vi "SelectSignals.vi"(8 "error in (no error)":errorcluster caption="Error in", 11 "DevicesAndSignals":T1) -> (0 "error out":errorcluster caption="Error out", 2 "Cancel":bool, 3 "DevicesAndSignals":T1)   [LabVIEW 2016]
doc: "Select certain signals that should be used later (e.g. for measuring).\n\nDevicesAndSignals (Input): Cluster consisting of an array of devices and an array of signals.\nDevicesAndSignals (Output): Cluster consisting of an array of devices and an array of SELECTED signals."
panel:
  in  "AdoptSelectedSignals":bool
  in  "Cancel":bool
  in  "tvAvailableSignals":string(tree)
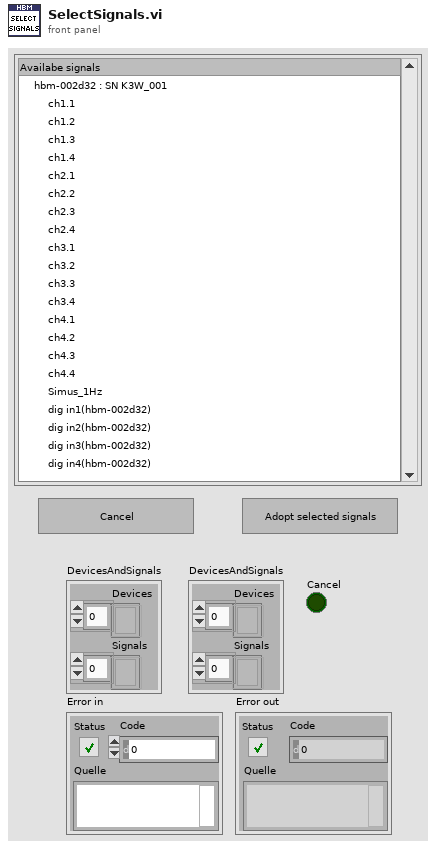
[diagram p1: front panel]
types:
  T1 = cluster{"Devices":refnum<k24>[], "Signals":refnum<k24>[]}
  T2 = typedef "LVPoint32TypeDef.ctl" = cluster{"Horizontal":i32, "Vertical":i32}
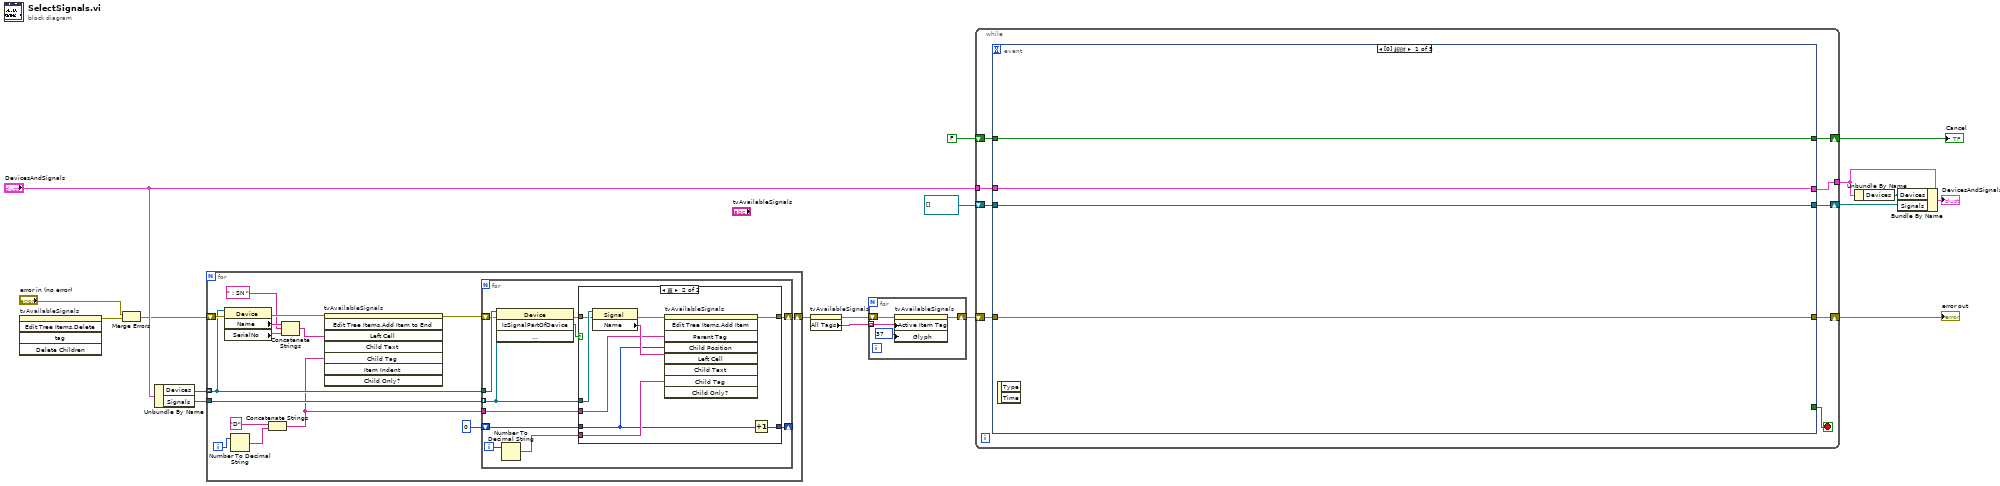
[diagram p0: block diagram]
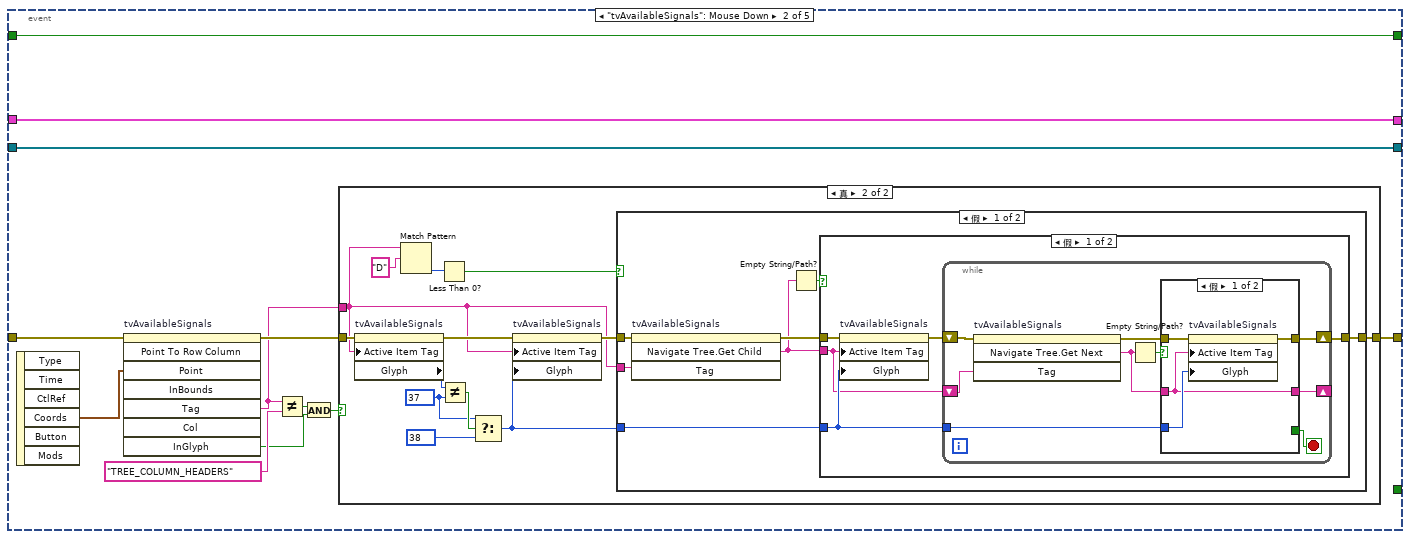
[diagram p3: hidden frame]
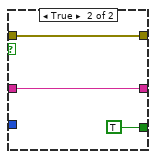
[diagram p5: hidden frame]
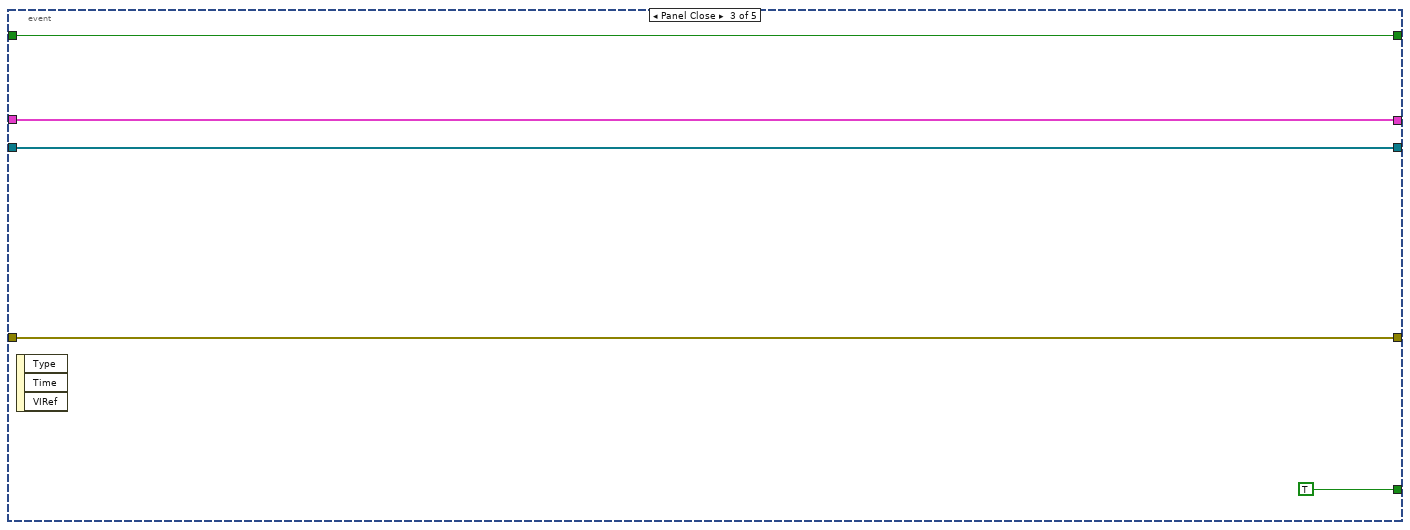
[diagram p8: hidden frame]
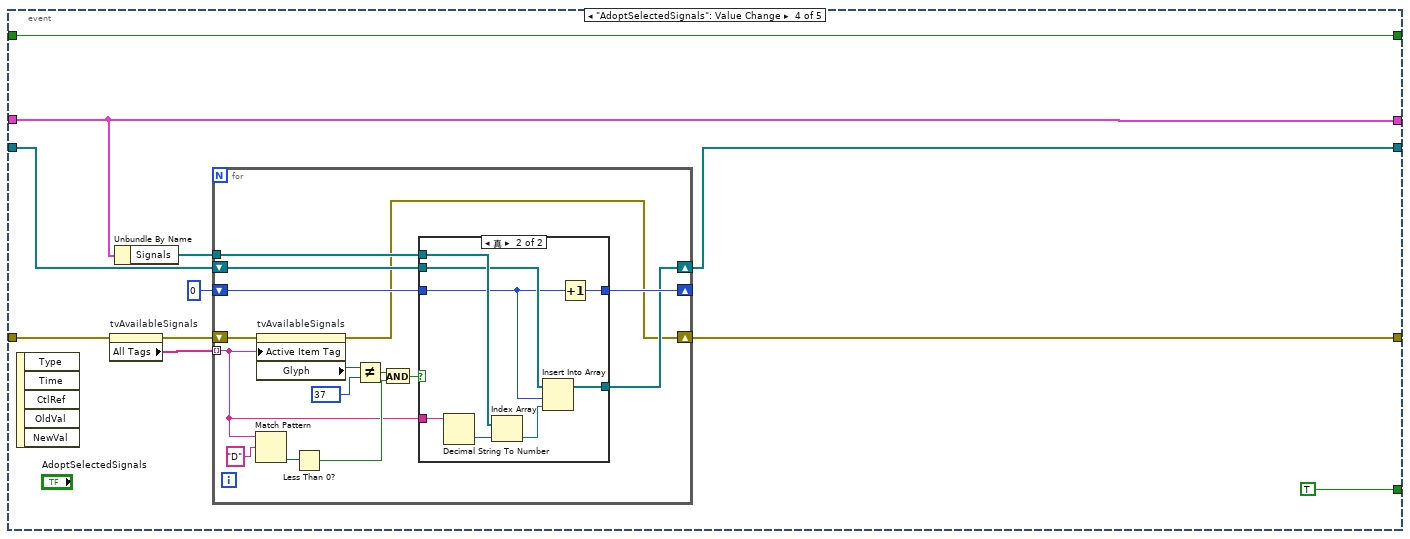
[diagram p9: hidden frame]
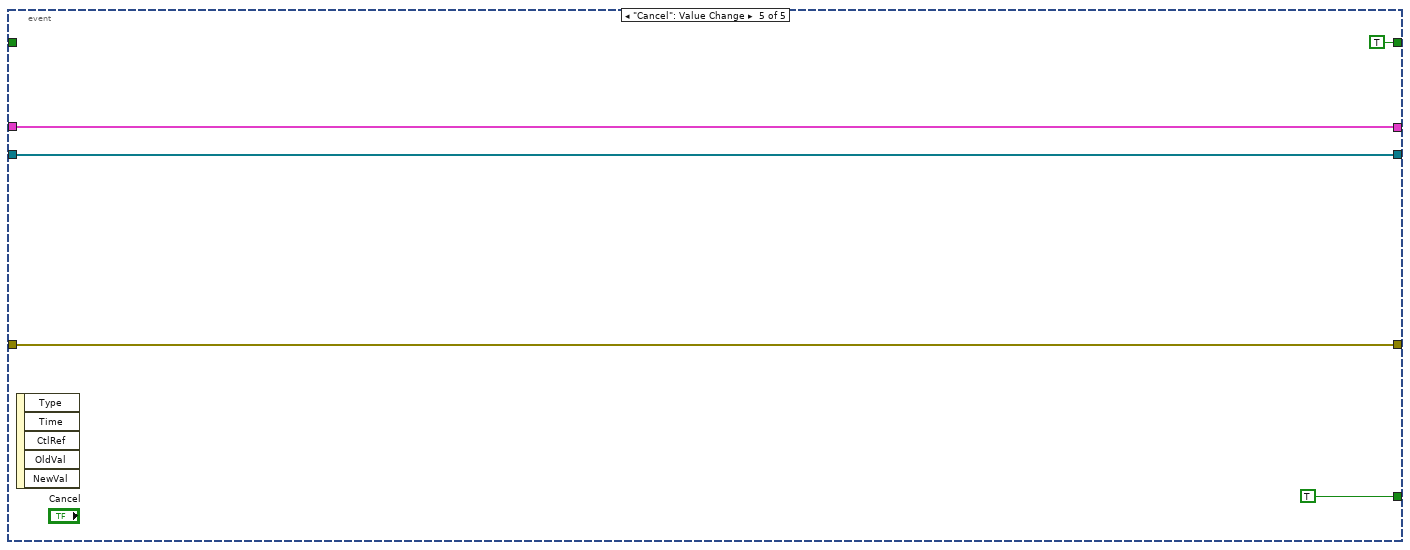
[diagram p11: hidden frame]
diagram:
  n1 = invoke on="tvAvailableSignals" class="Baum (strikt)" method="Edit Tree Items.Delete"() -> (error out=w5:errorcluster)  [unwired: 5 in, 4 out]
  n2 = Merge Errors("error in (no error)", w5) -> (w3:errorcluster)
  n3 = Unbundle By Name("DevicesAndSignals") -> ("Devices"=w14:refnum<k24>[], "Signals"=w13:refnum<k24>[])
  n4 = for {
    tunnel: w14 -> [w25] mode=indexing
    tunnel: w13 -> [w33]
    shift-right: [w19] -> w12
    shift-left: w3 -> [w31]
    i -> [w32]
    n5 = property on="Eigenschaftsknoten" class="Device"(reference=w25, error in=w31) -> (error out=w30:errorcluster, "Name"=w29:string, "SerialNo"=w28:string)  [unwired: 1 out]
    n6 = Number To Decimal String(number=w32) -> (decimal integer string=w23:string)  [unwired: 1 in]
    n7 = Concatenate Strings("D" ("String"), w23) -> (w22:string)
    n8 = Concatenate Strings(w29, " : SN " ("String"), w28) -> (w26:string)
    n9 = invoke on="tvAvailableSignals" class="Baum (strikt)" method="Edit Tree Items.Add Item to End"(error in=w30, "Left Cell"=w26, "Child Tag"=w22) -> (error out=w24:errorcluster)  [unwired: 5 in, 7 out]
    n10 = for {
      tunnel: w25 -> [w44]
      tunnel: w33 -> [w40] mode=indexing
      tunnel: w22 -> [w39]
      shift-right: [w35] -> _
      shift-left: 0 -> [w36]
      shift-right: [w34] -> w19
      shift-left: w24 -> [w42]
      i -> [w38]
      n11 = invoke on="Methodenknoten" class="Device" method="IsSignalPartOfDevice"(reference=w44, error in=w42, "signalToCheck"=w40) -> (error out=w41:errorcluster, "IsSignalPartOfDevice"=w43:bool)  [unwired: 1 in, 2 out]
      n12 = Number To Decimal String(number=w38) -> (decimal integer string=w37:string)  [unwired: 1 in]
      n13 = case shown="真" w43 {
        tunnel: w41 -> [w45 w54]
        tunnel: w40 -> [_ w55]
        tunnel: w39 -> [_ w51]
        tunnel: w37 -> [_ w50]
        tunnel: w36 -> [w46 w48]
        tunnel: [w46 w49] -> w35
        tunnel: [w45 w47] -> w34
        frame False {
        }
        frame True {
          n14 = property on="Eigenschaftsknoten" class="Signal"(reference=w55, error in=w54) -> (error out=w52:errorcluster, "Name"=w53:string)  [unwired: 1 out]
          n15 = invoke on="tvAvailableSignals" class="Baum (strikt)" method="Edit Tree Items.Add Item"(error in=w52, "Parent Tag"=w51, "Child Position"=w48, "Left Cell"=w53, "Child Tag"=w50) -> (error out=w47:errorcluster)  [unwired: 4 in, 8 out]
          n16 = Increment(x=w48) -> (x+1=w49:i32)
        }
      }
    }
  }
  n17 = property on="tvAvailableSignals" class="Tree (严格)"(error in=w12) -> (error out=w16:errorcluster, "All Tags"=w17:string[])  [unwired: 1 in, 1 out]
  n18 = for {
    tunnel: w17 -> [w59] mode=indexing
    shift-right: [w56] -> w15
    shift-left: w16 -> [w57]
    n19 = property on="tvAvailableSignals" class="Tree (严格)"(error in=w57, "Active Item Tag"=w59, "Glyph"=37) -> (error out=w56:errorcluster)  [unwired: 1 in, 1 out]
  }
  n20 = while {
    shift-right: [w66] -> w18
    shift-left: w15 -> [w67]
    shift-right: [w63] -> w7
    shift-left: refnum<k24>[] [] ("Signals") -> [w65]
    tunnel: "DevicesAndSignals" -> [w64]
    tunnel: [w62] -> w9
    shift-right: [w60] -> w1
    shift-left: FALSE -> [w61]
    stop <- w68 stop-if-true
    n21 = event shown="[0] 超时" {
      selector: _ -> [_ _ _ _ _]
      dyn-events: _ -> [_ _ _ _ _]
      timeout: _ -> [_ _ _ _ _]
      tunnel: [_ _ TRUE TRUE TRUE] -> w68
      tunnel: w67 -> [w72 w83 w130 w144 w173]
      tunnel: [w72 w81 w130 w136 w173] -> w66
      tunnel: w65 -> [w71 w74 w132 w141 w172]
      tunnel: w64 -> [w70 w75 w133 w140 w171]
      tunnel: [w70 w75 w133 w140 w171] -> w62
      tunnel: [w71 w74 w132 w137 w172] -> w63
      tunnel: w61 -> [w69 w73 w129 w134 _]
      tunnel: [w69 w73 w129 w134 TRUE] -> w60
      event Timeout {
        n22 = event-data() -> ()  [unwired: 1 in, 2 out]
      }
      event "tvAvailableSignals": Mouse Down {
        n23 = event-data() -> ("Coords"=w84:T2)  [unwired: 1 in, 5 out]
        n24 = invoke on="tvAvailableSignals" class="Baum (strikt)" method="Point To Row Column"(error in=w83, "Point"=w84) -> (error out=w82:errorcluster, "Tag"=w79:string, "InGlyph"=w76:bool)  [unwired: 6 in, 5 out]
        n25 = Not Equal?(x=w79, y="TREE_COLUMN_HEADERS") -> (x != y?=w77:bool)
        n26 = And(x=w77, y=w76) -> (x .and. y?=w78:bool)
        n27 = case shown="真" w78 {
          tunnel: w79 -> [_ w87]
          tunnel: w82 -> [w85 w95]
          tunnel: [w85 w93] -> w81
          frame False {
          }
          frame True {
            w96 = 37
            n28 = property on="tvAvailableSignals" class="Tree (严格)"(error in=w95, "Active Item Tag"=w87) -> (error out=w89:errorcluster, "Glyph"=w98:i32)  [unwired: 1 in, 1 out]
            n29 = Match Pattern(string=w87, regular expression="D" ("Format-String")) -> (offset past match=w91:i32)  [unwired: 1 in, 3 out]
            n30 = Less Than 0?(x=w91) -> (x < 0?=w90:bool)
            n31 = Not Equal?(x=w98, y=w96) -> (x != y?=w97:bool)
            n32 = Select(t=w96, s=w97, f=38) -> (s? t:f=w86:i32)
            n33 = property on="tvAvailableSignals" class="Tree (严格)"(error in=w89, "Active Item Tag"=w87, "Glyph"=w86) -> (error out=w88:errorcluster)  [unwired: 1 in, 1 out]
            n34 = case shown="假" w90 {
              tunnel: w88 -> [w101 w128]
              tunnel: w86 -> [w99 _]
              tunnel: [w103 w128] -> w93
              tunnel: w87 -> [w100 _]
              frame False {
                n35 = invoke on="tvAvailableSignals" class="Baum (strikt)" method="Navigate Tree.Get Child"(error in=w101, "Tag"=w100) -> (error out=w104:errorcluster, "Navigate Tree:Get Child"=w102:string)  [unwired: 2 in, 2 out]
                n36 = Empty String/Path?(string/path=w102) -> (empty?=w105:bool)
                n37 = case shown="假" w105 {
                  tunnel: w104 -> [w110 w127]
                  tunnel: [w109 w127] -> w103
                  tunnel: w99 -> [w107 _]
                  tunnel: w102 -> [w106 _]
                  frame False {
                    n38 = property on="tvAvailableSignals" class="Tree (严格)"(error in=w110, "Active Item Tag"=w106, "Glyph"=w107) -> (error out=w108:errorcluster)  [unwired: 1 in, 1 out]
                    n39 = while {
                      shift-right: [w114] -> w109
                      shift-left: w108 -> [w119]
                      tunnel: w107 -> [w113]
                      shift-right: [w111] -> _
                      shift-left: w106 -> [w116]
                      stop <- w117 stop-if-true
                      n40 = invoke on="tvAvailableSignals" class="Baum (strikt)" method="Navigate Tree.Get Next"(error in=w119, "Tag"=w116) -> (error out=w115:errorcluster, "Navigate Tree:Get Next Item"=w112:string)  [unwired: 2 in, 2 out]
                      n41 = Empty String/Path?(string/path=w112) -> (empty?=w118:bool)
                      n42 = case shown="假" w118 {
                        tunnel: [_ TRUE] -> w117
                        tunnel: w115 -> [w123 w125]
                        tunnel: [w122 w125] -> w114
                        tunnel: w113 -> [w121 _]
                        tunnel: w112 -> [w120 w124]
                        tunnel: [w120 w124] -> w111
                        frame False {
                          n43 = property on="tvAvailableSignals" class="Tree (严格)"(error in=w123, "Active Item Tag"=w120, "Glyph"=w121) -> (error out=w122:errorcluster)  [unwired: 1 in, 1 out]
                        }
                        frame True {
                        }
                      }
                    }
                  }
                  frame True {
                  }
                }
              }
              frame True {
              }
            }
          }
        }
      }
      event Panel Close {
        n44 = event-data() -> ()  [unwired: 1 in, 3 out]
      }
      event "AdoptSelectedSignals": Value Change {
        n45 = event-data() -> ()  [unwired: 1 in, 5 out]
        n46 = property on="tvAvailableSignals" class="Tree (严格)"(error in=w144) -> (error out=w142:errorcluster, "All Tags"=w143:string[])  [unwired: 1 in, 1 out]
        n47 = Unbundle By Name(w140) -> ("Signals"=w139:refnum<k24>[])
        n48 = for {
          tunnel: w143 -> [w151] mode=indexing
          shift-right: [w145] -> w136
          shift-left: w142 -> [w159]
          tunnel: w139 -> [w149]
          shift-right: [w147] -> _
          shift-left: 0 -> [w148]
          shift-right: [w146] -> w137
          shift-left: w141 -> [w150]
          n49 = Match Pattern(string=w151, regular expression="D" ("Format-String")) -> (offset past match=w155:i32)  [unwired: 1 in, 3 out]
          n50 = property on="tvAvailableSignals" class="Tree (严格)"(error in=w159, "Active Item Tag"=w151) -> (error out=w145:errorcluster, "Glyph"=w157:i32)  [unwired: 1 in, 1 out]
          n51 = Less Than 0?(x=w155) -> (x < 0?=w153:bool)
          n52 = Not Equal?(x=w157, y=37) -> (x != y?=w154:bool)
          n53 = And(x=w154, y=w153) -> (x .and. y?=w152:bool)
          n54 = case shown="真" w152 {
            tunnel: w151 -> [_ w169]
            tunnel: w149 -> [_ w167]
            tunnel: w150 -> [w160 w166]
            tunnel: [w160 w165] -> w146
            tunnel: w148 -> [w161 w163]
            tunnel: [w161 w162] -> w147
            frame False {
            }
            frame True {
              n55 = Decimal String To Number(string=w169) -> (number=w168:i32)  [unwired: 2 in, 1 out]
              n56 = Index Array(array=w167, index=w168) -> (element=w164:refnum<k24>)
              n57 = Insert Into Array(array=w166, index=w163, new element=w164) -> (w165:refnum<k24>[])
              n58 = Increment(x=w163) -> (x+1=w162:i32)
            }
          }
        }
      }
      event "Cancel": Value Change {
        n59 = event-data() -> ()  [unwired: 1 in, 5 out]
      }
    }
  }
  "error out" <- w18
  "Cancel" <- w1
  n60 = Unbundle By Name(w9) -> ("Devices"=w8:refnum<k24>[])
  n61 = Bundle By Name(cluster=w9, "Devices"=w8, "Signals"=w7) -> (→"DevicesAndSignals":T1)
